vi "VIA Per VI Results.vi"(7 "Root Dir":path, 8 "Error in":errorcluster caption="Error in (no error)", 10 "Ranking Thresholds":T1={"High"=100.0, "Normal"=90.0, "Low"=80.0}, 11 "VIAResult":T10 {"Test Config Data"."Test Ranking" items=["Low", "Normal", "High"]}) -> (0 "Error out":errorcluster, 1 "Per VI Ranking CSV String":string, 2 "Pass?":bool, 3 "Per VI Results String":string)   [LabVIEW 2023, in "VIA Results Handling.lvlib"]
doc: "Takes in VIA Results, Ranking Thresholds, and a Root Directory to determine pass/fail.\nOutputs a Per VI Results String and CSV String."
uses:
  VIA Results Handling.lvlib
  <vilib>/addons/analyzer/_analyzerctrls.llb/VIAnCtl Results.ctl
  <vilib>/addons/analyzer/_analyzerctrls.llb/VIAnCtl ResultsData (index).ctl
  <vilib>/addons/analyzer/_analyzerctrls.llb/VIAnCtl ResultStatus.ctl
  <vilib>/addons/analyzer/_vianresshared.llb/VIAnRes Parsed Results Data (by VI).ctl
  <vilib>/addons/analyzer/_vianresshared.llb/VIAnRes Parsed Results Data (by Test).ctl
  <vilib>/addons/analyzer/_analyzerctrls.llb/VIAnCtl Test Config Data.ctl
  <vilib>/addons/analyzer/_analyzerctrls.llb/VIAnCtl TestRanking.ctl
  <vilib>/addons/analyzer/_analyzerctrls.llb/VIAnCtl Config Control Value.ctl
  Ranking Thresholds.ctl
  Stats by Ranking.ctl
  Stats Cluster.ctl
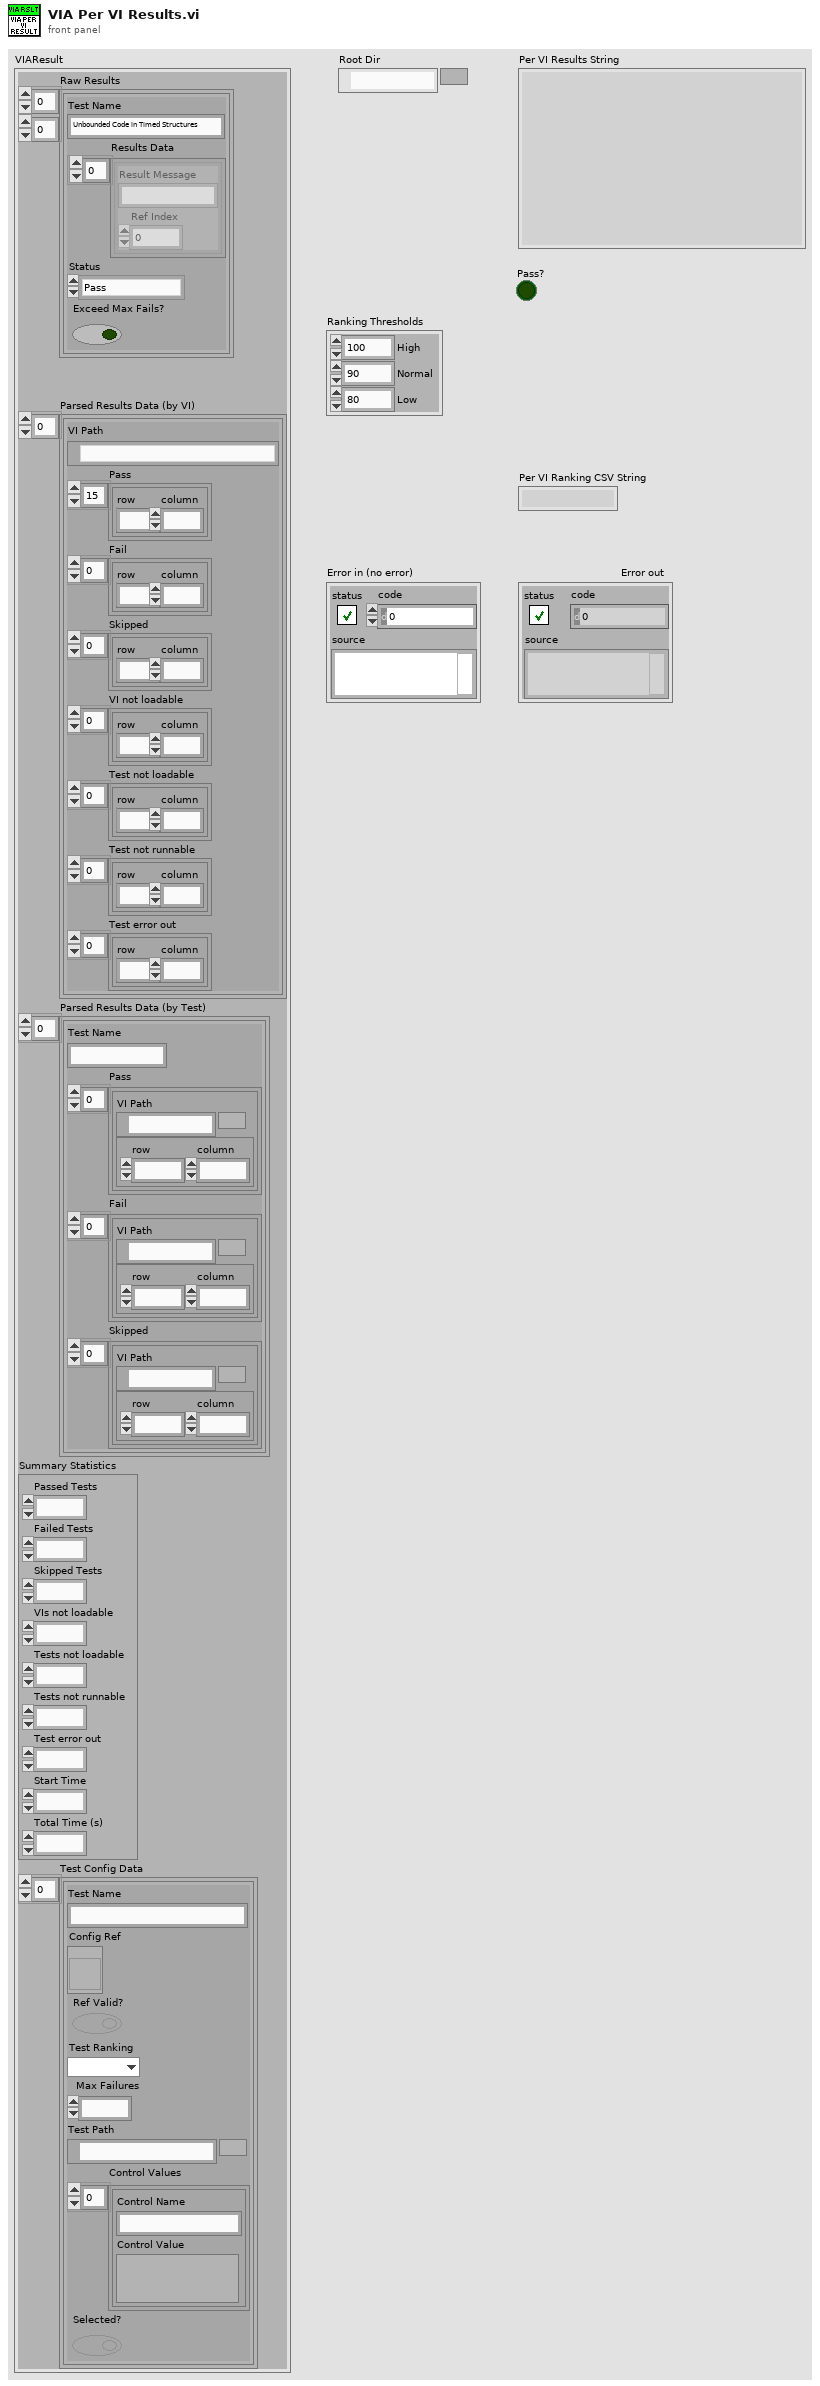
[diagram p1: front panel]
types:
  T1 = typedef "VIA Results Handling.lvlib/Ranking Thresholds.ctl" = cluster{"High":dbl, "Normal":dbl, "Low":dbl}
  T2 = typedef "VIAnCtl Results.ctl" = cluster{"Test Name":string, "Results Data":T3[], "Status":T4, "Exceed Max Fails?":bool}
  T3 = typedef "VIAnCtl ResultsData (index).ctl" = cluster{"Result Message":string, "Ref Index":i32}
  T4 = typedef "VIAnCtl ResultStatus.ctl" = enum16{"Pass", "Fail", "Skipped", "VI not loadable", "Test not loadable", "Test not runnable", "Test error out"}
  T5 = typedef "VIAnRes Parsed Results Data (by VI).ctl" = cluster{"VI Path":path, "Pass":cluster{"row":i32, "column":i32}[], "Fail":cluster{"row":i32, "column":i32}[], "Skipped":cluster{"row":i32, "column":i32}[], "VI not loadable":cluster{"row":i32, "column":i32}[], "Test not loadable":cluster{"row":i32, "column":i32}[], "Test not runnable":cluster{"row":i32, "column":i32}[], "Test error out":cluster{"row":i32, "column":i32}[]}
  T6 = typedef "VIAnRes Parsed Results Data (by Test).ctl" = cluster{"Test Name":string, "Pass":cluster{"VI Path":path, "index":cluster{"row":i32, "column":i32}}[], "Fail":cluster{"VI Path":path, "index":cluster{"row":i32, "column":i32}}[], "Skipped":cluster{"VI Path":path, "index":cluster{"row":i32, "column":i32}}[]}
  T7 = typedef "VIAnCtl Test Config Data.ctl" = cluster{"Test Name":string, "Config Ref":refnum<vi>, "Ref Valid?":bool, "Test Ranking":T8, "Max Failures":u32, "Test Path":path, "Control Values":T9[], "Selected?":bool}
  T8 = typedef "VIAnCtl TestRanking.ctl" = u16
  T9 = typedef "VIAnCtl Config Control Value.ctl" = cluster{"Control Name":string, "Control Value":variant}
  T10 = cluster{"Raw Results":T2[][], "Parsed Results Data (by VI)":T5[], "Parsed Results Data (by Test)":T6[], "Summary Statistics":cluster{"Passed Tests":i32, "Failed Tests":i32, "Skipped Tests":i32, "VIs not loadable":i32, "Tests not loadable":i32, "Tests not runnable":i32, "Test error out":i32, "Start Time":u32, "Total Time (s)":dbl}, "Test Config Data":T7[]}
  T11 = typedef "VIA Results Handling.lvlib/Stats by Ranking.ctl" = cluster{"High":T12, "Normal":T12, "Low":T12}
  T12 = typedef "VIA Results Handling.lvlib/Stats Cluster.ctl" = cluster{"Passed":i32, "Failed":i32, "Skipped":i32, "Total":i32}
  T13 = typedef "VIA Results Handling.lvlib/Ranking Percent Passing Cluster.ctl" = cluster{"High":dbl, "Normal":dbl, "Low":dbl}
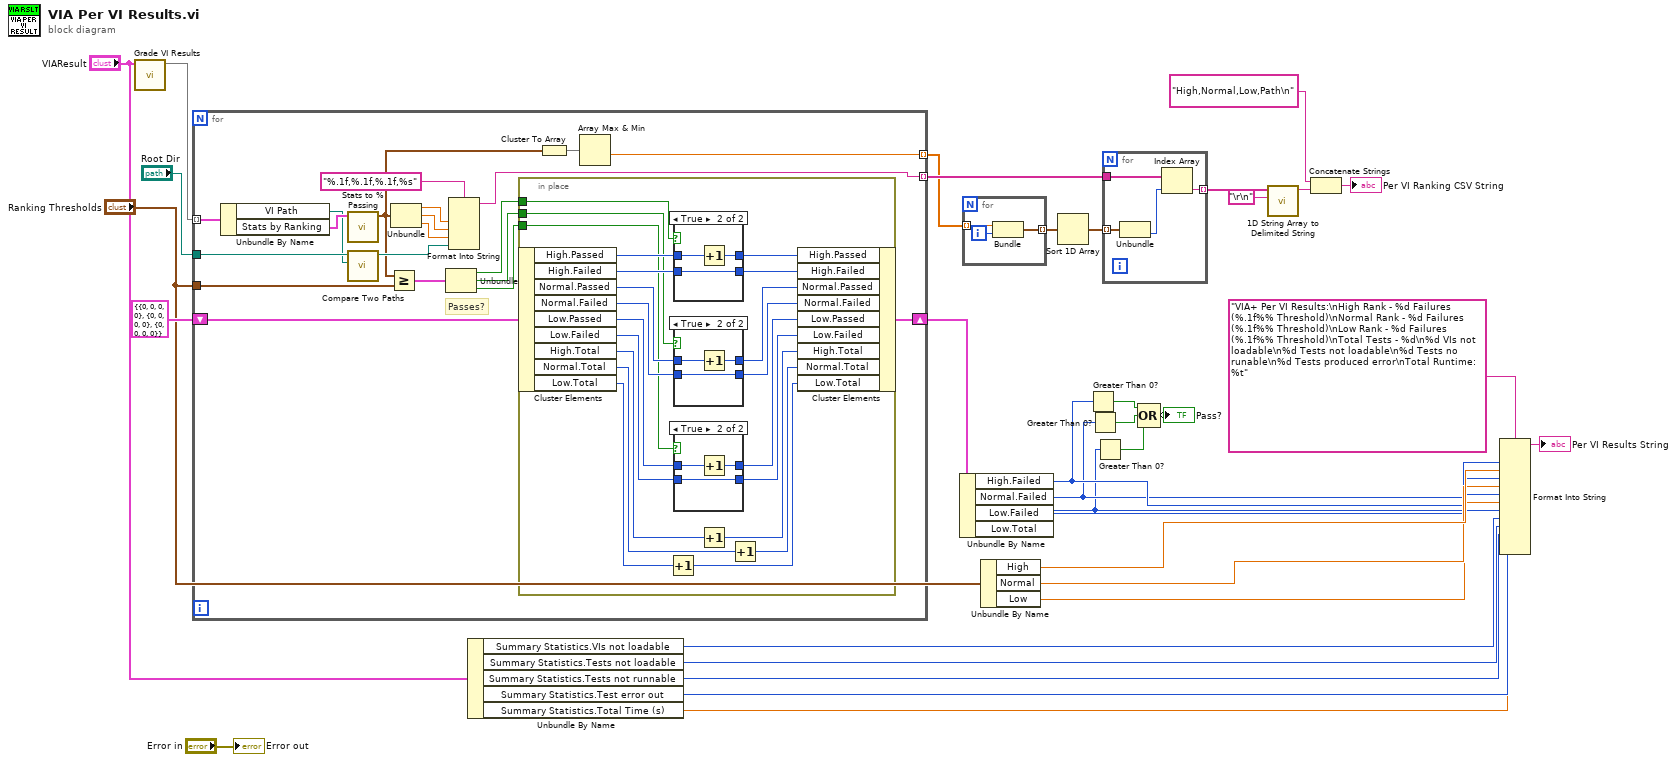
[diagram p0: block diagram]
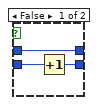
[diagram p2: hidden frame]
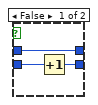
[diagram p3: hidden frame]
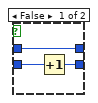
[diagram p4: hidden frame]
diagram:
  n1 = call "Grade VI Results.vi"("VIAResult"="VIAResult") -> ("VI Stats Map"=w34:map{path, T11})  [unwired: 9 in, 1 out]
  n2 = for {
    tunnel: w34 -> [w54] mode=indexing
    tunnel: "Root Dir" -> [w52]
    tunnel: [w46] -> w4 mode=indexing
    tunnel: "Ranking Thresholds" -> [w44]
    shift-right: [w41] -> w24
    shift-left: T11 {"High"={"Passed"=0, "Failed"=0, "Skipped"=0, "Total"=0}, "Normal"={"Passed"=0, "Failed"=0, "Skipped"=0, "Total"=0}, "Low"={"Passed"=0, "Failed"=0, "Skipped"=0, "Total"=0}} ("Stats by Ranking") -> [w42]
    tunnel: [w35] -> w2 mode=indexing
    # "Passes?"
    n3 = Unbundle By Name(w54) -> ("VI Path"=w51:path, "Stats by Ranking"=w53:T11)
    n4 = call "Stats to % Passing.vi"("Stats by Ranking"=w53) -> ("% Passing"=w37:T13)  [unwired: 10 in]
    n5 = call <vilib>:"Compare Two Paths.vi"("Path 2"=w51, "Path 1"=w52) -> ("Relative Path from 1 to 2"=w47:path)  [unwired: 6 in, 3 out]
    n6 = Greater Or Equal?(x=w37, y=w44) -> (x >= y?=w43:cluster{"High":bool, "Normal":bool, "Low":bool})
    n7 = Unbundle(w37) -> ("High"=w45:dbl, "Normal"=w49:dbl, "Low"=w48:dbl)
    n8 = Unbundle(w43) -> ("High"=w40:bool, "Normal"=w39:bool, "Low"=w38:bool)
    n9 = Format Into String(format string="%.1f,%.1f,%.1f,%s", w45, w49, w48, w47) -> (resulting string=w46:string)  [unwired: 2 in, 1 out]
    n10 = in-place {
      in-place-border: w40 -> [w67]
      in-place-border: w39 -> [w61]
      in-place-border: w38 -> [w55]
      n11 = in-place-cluster #1(w42) -> ("High.Passed"=w70:i32, "High.Failed"=w68:i32, "Normal.Passed"=w64:i32, "Normal.Failed"=w65:i32, "Low.Passed"=w59:i32, "Low.Failed"=w58:i32, "High.Total"=w75:i32, "Normal.Total"=w74:i32, "Low.Total"=w73:i32)
      n12 = Increment(x=w73) -> (x+1=w60:i32)
      n13 = case shown="True" w67 {
        tunnel: [w90 w91] -> w71
        tunnel: w70 -> [w90 w93]
        tunnel: [w88 w92] -> w69
        tunnel: w68 -> [w89 w92]
        frame False {
          n14 = Increment(x=w89) -> (x+1=w88:i32)
        }
        frame True {
          n15 = Increment(x=w93) -> (x+1=w91:i32)
        }
      }
      n16 = case shown="True" w61 {
        tunnel: [w84 w85] -> w63
        tunnel: w64 -> [w84 w87]
        tunnel: [w82 w86] -> w62
        tunnel: w65 -> [w83 w86]
        frame False {
          n17 = Increment(x=w83) -> (x+1=w82:i32)
        }
        frame True {
          n18 = Increment(x=w87) -> (x+1=w85:i32)
        }
      }
      n19 = case shown="True" w55 {
        tunnel: [w78 w79] -> w57
        tunnel: w59 -> [w78 w81]
        tunnel: [w76 w80] -> w56
        tunnel: w58 -> [w77 w80]
        frame False {
          n20 = Increment(x=w77) -> (x+1=w76:i32)
        }
        frame True {
          n21 = Increment(x=w81) -> (x+1=w79:i32)
        }
      }
      n22 = Increment(x=w75) -> (x+1=w66:i32)
      n23 = Increment(x=w74) -> (x+1=w72:i32)
      n24 = in-place-cluster #1("High.Passed"=w71, "High.Failed"=w69, "Normal.Passed"=w63, "Normal.Failed"=w62, "Low.Passed"=w57, "Low.Failed"=w56, "High.Total"=w66, "Normal.Total"=w72, "Low.Total"=w60) -> (w41:T11)
    }
    n25 = Cluster To Array(cluster=w37) -> (array=w36:dbl[])
    n26 = Array Max & Min(array=w36) -> (min value=w35:dbl)  [unwired: 3 out]
  }
  n27 = Unbundle By Name("VIAResult") -> ("Summary Statistics.VIs not loadable"=w18:i32, "Summary Statistics.Tests not loadable"=w17:i32, "Summary Statistics.Tests not runnable"=w16:i32, "Summary Statistics.Test error out"=w15:i32, "Summary Statistics.Total Time (s)"=w14:dbl)
  n28 = Unbundle By Name(w24) -> ("High.Failed"=w12:i32, "Normal.Failed"=w11:i32, "Low.Failed"=w20:i32, "Low.Total"=w10:i32)
  n29 = for {
    tunnel: w2 -> [w96] mode=indexing
    tunnel: [w94] -> w3 mode=indexing
    i -> [w95]
    n30 = Bundle(w96, w95) -> (w94:cluster{dbl, i32})  [unwired: 1 in]
  }
  n31 = Unbundle By Name("Ranking Thresholds") -> ("High"=w22:dbl, "Normal"=w21:dbl, "Low"=w19:dbl)
  n32 = Sort 1D Array(array=w3) -> (sorted array=w1:cluster{dbl, i32}[])
  n33 = Greater Than 0?(x=w12) -> (x > 0?=w9:bool)
  n34 = Greater Than 0?(x=w11) -> (x > 0?=w8:bool)
  n35 = Greater Than 0?(x=w10) -> (x > 0?=w7:bool)
  n36 = for {
    tunnel: w4 -> [w100]
    tunnel: [w99] -> w5 mode=indexing
    tunnel: w1 -> [w98] mode=indexing
    n37 = Unbundle(w98) -> (w97:i32)  [unwired: 1 out]
    n38 = Index Array(array=w100, index=w97) -> (element=w99:string)
  }
  n39 = Compound Arithmetic op=OR(w9, w8, w7) -> (invert →"Pass?":bool)
  n40 = call <vilib>:"1D String Array to Delimited String.vi"("delimiter"="\r\n", "string array"=w5) -> ("delimited string"=w32:string)  [unwired: 9 in]
  n41 = Concatenate Strings("High,Normal,Low,Path\n" ("format string"), w32) -> (→"Per VI Ranking CSV String":string)
  n42 = Format Into String(format string="VIA+ Per VI Results:\nHigh Rank - %d Failures (%.1f%% Threshold)\nNormal Rank - %d Failures (%.1f%% Threshold)\nLow Rank - %d Failures (%.1f%% Threshold)\nTotal Tests - %d\n%d VIs not loadable\n%d Tests not loadable\n%d Tests no runable\n%d Tests produced error\nTotal Runtime: %t", w12, w22, w11, w21, w20, w19, w10, w18, w17, w16, w15, w14) -> (resulting string=→"Per VI Results String":string)  [unwired: 2 in, 1 out]
  "Error out" <- "Error in"
